vi "Example_5207.vi"() -> ()   [LabVIEW 2015]
panel:
  out "Gauge":dbl(knob) scale=0.0..10.0
  out "Numeric":dbl
  out "Waveform Chart":dbl(graph)
  in  "stop":bool
  in  "Sensitivity (mV)":dbl
  in  "error in (no error)":errorcluster
  in  "VISA resource name":refnum<visa-resource-name>
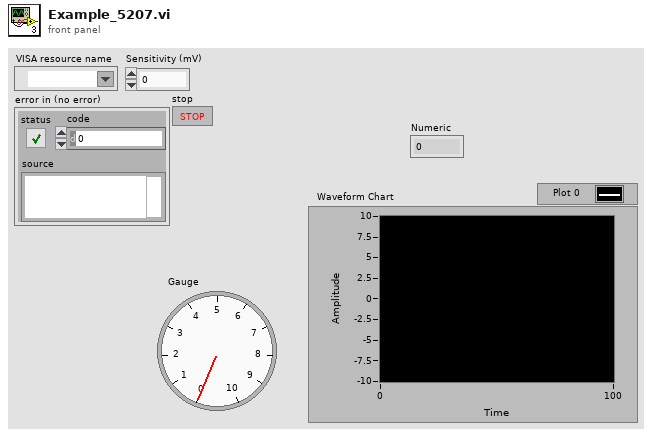
[diagram p1: front panel]
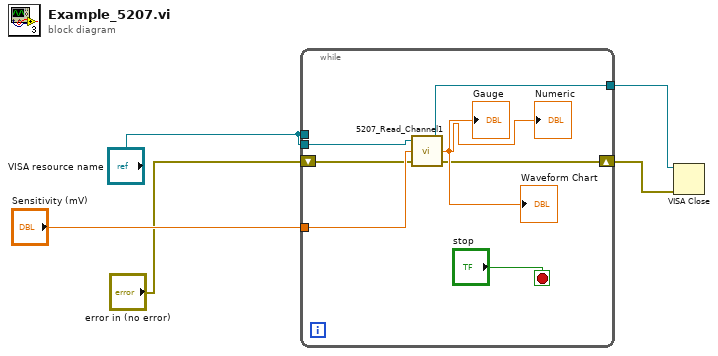
[diagram p0: block diagram]
diagram:
  n1 = while {
    tunnel: "VISA resource name" -> [_]
    tunnel: "VISA resource name" -> [w11]
    tunnel: "Sensitivity (mV)" -> [w10]
    tunnel: [w7] -> w3
    shift-right: [w8] -> w2
    shift-left: "error in (no error)" -> [w6]
    stop <- "stop" stop-if-true
    n2 = call "5207_Read_Channel1.vi"("error in (no error)"=w6, "Sensitivity (mV)"=w10, "VISA resource name"=w11) -> ("error out"=w8:errorcluster, "Channel 1"=→"Waveform Chart" →"Gauge" →"Numeric":dbl, "VISA resource name out"=w7:refnum<visa-resource-name>)
  }
  n3 = VISA Close(VISA resource name=w3, error in (no error)=w2) -> ()  [unwired: 1 out]
